vi "TrajectoryState_AlmostEquals.vi"(6 "Tolerance":dbl=1e-05 format="%#_13g", 9 "Other TRAJ_STATE":T1={"TimeSeconds"=0.0, "Velocity"=0.0, "Acceleration"=0.0, "POSE"={"TRANSLATION"={"X"=0.0, "Y"=0.0}, "ROTATION"={"VALUE"=0.0, "COS"=1.0, "SIN"=0.0}}, "Curvature"=0.0} {"POSE"."ROTATION"."SIN" format="%13.4f"; "POSE"."ROTATION"."COS" format="%13.4f"; "POSE"."ROTATION"."VALUE" format="%13.4f"; "POSE"."TRANSLATION"."Y" format="%14.3f"; "POSE"."TRANSLATION"."X" format="%14.3f"}, 11 "TRAJ_STATE":T1={"TimeSeconds"=0.0, "Velocity"=0.0, "Acceleration"=0.0, "POSE"={"TRANSLATION"={"X"=0.0, "Y"=0.0}, "ROTATION"={"VALUE"=0.0, "COS"=1.0, "SIN"=0.0}}, "Curvature"=0.0} {"POSE"."ROTATION"."SIN" format="%13.4f"; "POSE"."ROTATION"."COS" format="%13.4f"; "POSE"."ROTATION"."VALUE" format="%13.4f"; "POSE"."TRANSLATION"."Y" format="%14.3f"; "POSE"."TRANSLATION"."X" format="%14.3f"}) -> (3 "Equals":bool)   [LabVIEW 2019]
doc: "Determines if two Trajectory States are equal\n \nParameters:\n - TrajState - TrajectoryState data structure\n - Other TrajState - Other TrajectoryState data structure\n \nReturns:\n - Equals - boolean indicating if the states are equal."
uses:
  <vilib>/Rock Robotics/WPI/ThirdParty/JAS_Junk/TrajLib/TRAJ_STATE.ctl
  <vilib>/Rock Robotics/WPI/ThirdParty/JAS_Junk/TrajLib/POSE2D.ctl
  <vilib>/Rock Robotics/WPI/ThirdParty/JAS_Junk/TrajLib/TRANSLATION2D.ctl
  <vilib>/Rock Robotics/WPI/ThirdParty/JAS_Junk/TrajLib/ROTATION2D.ctl
  Translation_AlmostEquals.vi
  Rotation_AlmostEquals.vi
  <vilib>/Rock Robotics/WPI/ThirdParty/JAS_Junk/TrajLib/Util_CalcDist.vi
  <vilib>/Rock Robotics/WPI/ThirdParty/JAS_Junk/TrajLib/Trajectory_Library.lvlib
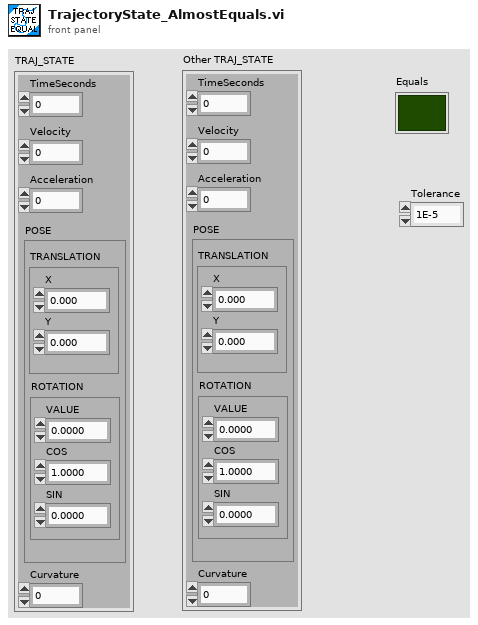
[diagram p1: front panel]
types:
  T1 = typedef "Trajectory_Library.lvlib/TRAJ_STATE.ctl" = cluster{"TimeSeconds":dbl, "Velocity":dbl, "Acceleration":dbl, "POSE":T2, "Curvature":dbl}
  T2 = typedef "Trajectory_Library.lvlib/POSE2D.ctl" = cluster{"TRANSLATION":T3, "ROTATION":T4}
  T3 = typedef "Trajectory_Library.lvlib/TRANSLATION2D.ctl" = cluster{"X":dbl, "Y":dbl}
  T4 = typedef "Trajectory_Library.lvlib/ROTATION2D.ctl" = cluster{"VALUE":dbl, "COS":dbl, "SIN":dbl}
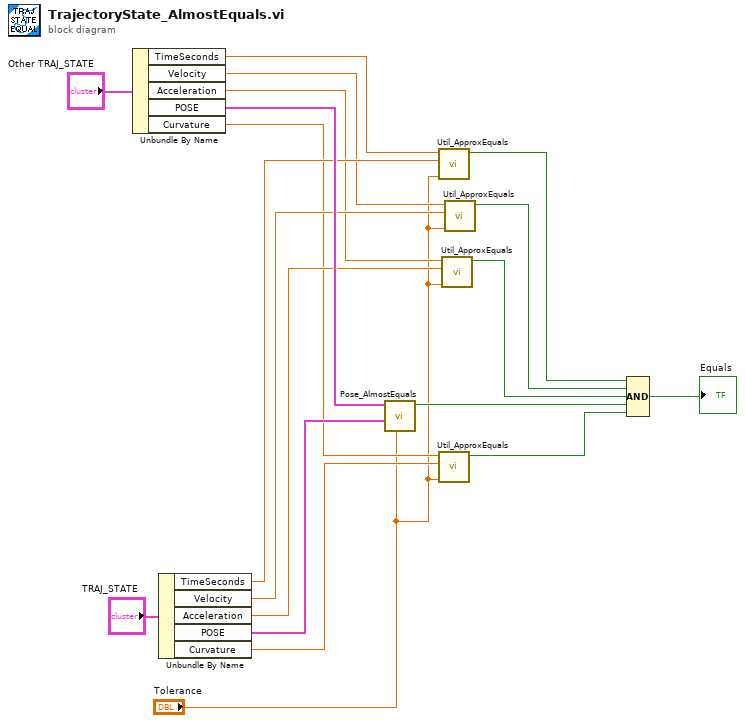
[diagram p0: block diagram]
diagram:
  n1 = Unbundle By Name("Other TRAJ_STATE") -> ("TimeSeconds"=w13:dbl, "Velocity"=w10:dbl, "Acceleration"=w7:dbl, "POSE"=w17:T2, "Curvature"=w4:dbl)
  n2 = Unbundle By Name("TRAJ_STATE") -> ("TimeSeconds"=w12:dbl, "Velocity"=w9:dbl, "Acceleration"=w6:dbl, "POSE"=w16:T2, "Curvature"=w3:dbl)
  n3 = call "Pose_AlmostEquals.vi"("Tolerance"="Tolerance", "other POSE"=w16, "in POSE"=w17) -> ("Equals"=w15:bool)  [unwired: 8 in]
  n4 = call <vilib>:"Util_ApproxEquals.vi"("Tolerance"="Tolerance", "Value 2"=w12, "Value 1"=w13) -> ("ApproxEquals"=w11:bool)  [unwired: 8 in]
  n5 = call <vilib>:"Util_ApproxEquals.vi"("Tolerance"="Tolerance", "Value 2"=w3, "Value 1"=w4) -> ("ApproxEquals"=w2:bool)  [unwired: 8 in]
  n6 = call <vilib>:"Util_ApproxEquals.vi"("Tolerance"="Tolerance", "Value 2"=w6, "Value 1"=w7) -> ("ApproxEquals"=w5:bool)  [unwired: 8 in]
  n7 = call <vilib>:"Util_ApproxEquals.vi"("Tolerance"="Tolerance", "Value 2"=w9, "Value 1"=w10) -> ("ApproxEquals"=w8:bool)  [unwired: 8 in]
  n8 = Compound Arithmetic op=AND(w11, w8, w5, w15, w2) -> (→"Equals":bool)
